vi "KG&KA.vi"(10 "Accelerometer range":enum16{"2", "4", "6", "8", "10", "15", "40"}(ring), 11 "Gyro rande":T1(ring)) -> (2 "KA":i32, 3 "KG":i32)   [LabVIEW 2017, in "IL Driver Library.lvlib"]
uses:
  IL Driver Library.lvlib
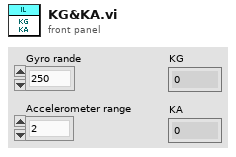
[diagram p1: front panel]
types:
  T1 = enum16{"250", "300", "450", "500", "1000", "2000"}
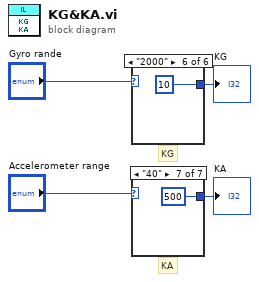
[diagram p0: block diagram]
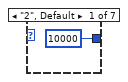
[diagram p2: hidden frame]
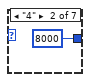
[diagram p3: hidden frame]
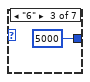
[diagram p4: hidden frame]
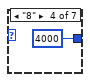
[diagram p5: hidden frame]
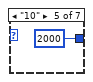
[diagram p6: hidden frame]
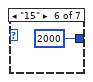
[diagram p7: hidden frame]
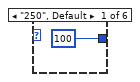
[diagram p8: hidden frame]
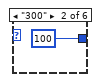
[diagram p9: hidden frame]
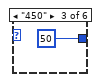
[diagram p10: hidden frame]
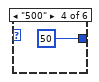
[diagram p11: hidden frame]
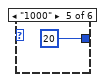
[diagram p12: hidden frame]
diagram:
  # "KA"
  # "KG"
  n1 = case shown="\"2000\"" "Gyro rande" {
    tunnel: [100 100 50 50 20 10] -> w4
    frame "250", Default {
    }
    frame "300" {
    }
    frame "450" {
    }
    frame "500" {
    }
    frame "1000" {
    }
    frame "2000" {
    }
  }
  "KG" <- w4
  n2 = case shown="\"40\"" "Accelerometer range" {
    tunnel: [10000 8000 5000 4000 2000 2000 500] -> w3
    frame "2", Default {
    }
    frame "4" {
    }
    frame "6" {
    }
    frame "8" {
    }
    frame "10" {
    }
    frame "15" {
    }
    frame "40" {
    }
  }
  "KA" <- w3
